vi "SubVI_BinDivider.vi"(1 "Spike Times":dbl[](array[numeric]), 2 "Total Duration [ms]":i32, 3 "Number of Bins":i32) -> (0 "Array":bool[](array[boolean]))   [LabVIEW 2018]
panel:
  out "Bin Duration":dbl
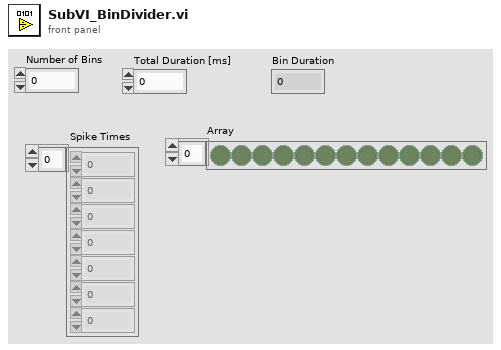
[diagram p1: front panel]
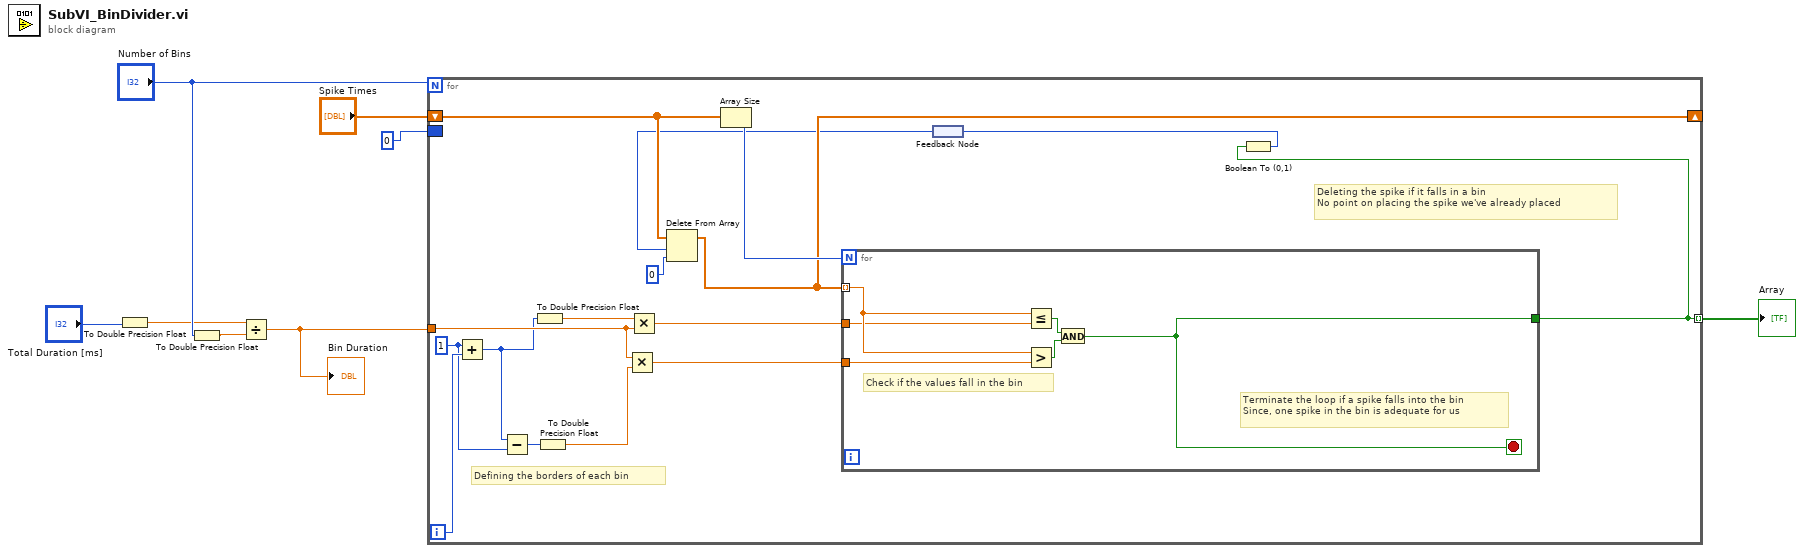
[diagram p0: block diagram]
diagram:
  n1 = To Double Precision Float(number="Total Duration [ms]") -> (double precision float=w2:dbl)
  n2 = To Double Precision Float(number="Number of Bins") -> (double precision float=w6:dbl)
  n3 = Divide(x=w2, y=w6) -> (x/y=w7:dbl)
  "Bin Duration" <- w7
  n4 = for {
    N: "Number of Bins" -> [_]
    tunnel: w7 -> [w18]
    tunnel: [w13] -> w8 mode=indexing
    shift-right: [w10] -> _
    shift-left: "Spike Times" -> [w11]
    border: i16 0 -> [_]
    i -> [w21]
    w15 = 1 ("y")
    # "Deleting the spike if it falls in a bin\nNo point on placing the spike we've already placed"
    # "Defining the borders of each bin"
    n5 = Add(x=w15, y=w21) -> (x+y=w16:i32)
    n6 = Subtract(x=w16, y=w15) -> (x-y=w20:i32)
    n7 = To Double Precision Float(number=w16) -> (double precision float=w23:dbl)
    n8 = To Double Precision Float(number=w20) -> (double precision float=w19:dbl)
    n9 = Multiply(x=w18, y=w19) -> (x*y=w17:dbl)
    n10 = Multiply(x=w23, y=w18) -> (x*y=w22:dbl)
    n11 = Array Size(array=w11) -> (size(s)=w24:i32)
    n12 = feedback #1() -> (w9:i16)
    n13 = Delete From Array(array=w11, length=w9, index=0) -> (array with subset deleted=w10:dbl[])  [unwired: 1 out]
    n14 = for {
      N: w24 -> [_]
      tunnel: w10 -> [w30] mode=indexing
      tunnel: w22 -> [w27]
      tunnel: [w25] -> w13
      tunnel: w17 -> [w26]
      stop <- w25 stop-if-true
      # "Terminate the loop if a spike falls into the bin\nSince, one spike in the bin is adequate for us"
      # "Check if the values fall in the bin"
      n15 = Less Or Equal?(x=w30, y=w27) -> (x <= y?=w28:bool)
      n16 = Greater?(x=w30, y=w26) -> (0:w29:bool)
      n17 = And(x=w28, y=w29) -> (x .and. y?=w25:bool)
    }
    n18 = Boolean To (0,1)(Boolean=w13) -> (0, 1=w12:i16)
    n19 = feedback-in #1(w12) -> ()
  }
  "Array" <- w8
